vi "usb relay init.vi"(8 "error in (no error)":errorcluster caption="entrée d'erreur (pas d'erreur)") -> (0 "error out":errorcluster caption="sortie d'erreur")   [LabVIEW 2020, in "usb_relay_device.lvlib"]
doc: "int EXPORT_API usb_relay_init(void);"
uses:
  usb_relay_device.lvlib
  usb_relay_device.dll
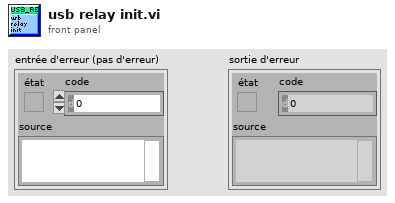
[diagram p1: front panel]
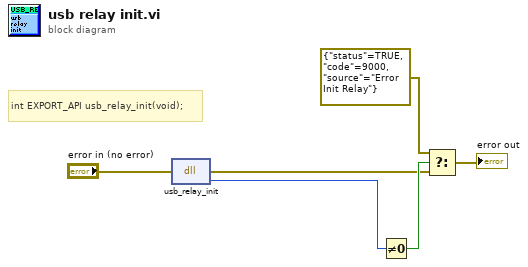
[diagram p0: block diagram]
diagram:
  # "int EXPORT_API usb_relay_init(void);"
  n1 = dll-call lib="C:/Users/ngarcin/OneDrive - Altyor/Standard TB/Class/Relay_Board/Relay_Board usb_Relay_device/usb_relay_device/usb_relay_device.*" fn="usb_relay_init"(error in="error in (no error)") -> (error out=w3:errorcluster, w4:i32)  [unwired: 2 in, 1 out]
  n2 = Not Equal To 0?(x=w4) -> (x != 0?=w5:bool)
  n3 = Select(t=errorcluster {"status"=TRUE, "code"=9000, "source"="Error Init Relay"} ("sortie d'erreur"), s=w5, f=w3) -> (s? t:f=→"error out":errorcluster)
